vi "FTW-JSON-Variant-Serialize.vi"(0 "Variant":variant, 9 "Pretty Print":bool=TRUE, 11 "error in":errorcluster) -> (4 "JSON String":string, 15 "error out":errorcluster)   [LabVIEW 2015]
uses:
  <vilib>/Utility/Data Type/NI_Data Type.lvlib
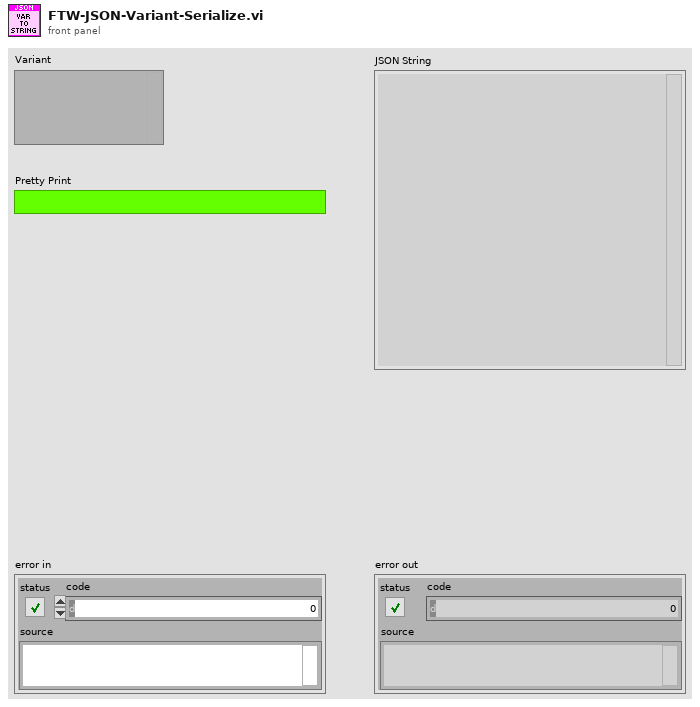
[diagram p1: front panel]
types:
  T1 = cluster{"Include Name":bool, "Indent":i32, "Spaces":i32, "Pretty Print":bool}
  T2 = typedef "NI_Data Type.lvlib/Data Type.ctl" = enum8{"Invalid Type", "Void", "I8", "I16", "I32", "I64", "U8", "U16", "U32", "U64", "Single Float", "Double Float", "Extended Float", "Single Complex", "Double Complex", "Extended Complex", "Enum U8", "Enum U16", "Enum U32", "Enum U64", "Single Float With Unit", "Double Float With Unit", "Extended Float With Unit", "Single Complex with Unit", "Double Complex with Unit", "Extended Complex with Unit", "Boolean", "String", "Path", "Picture", "Tag", "Array", "Cluster", "Variant", "LV Variant", "Waveform", "Timestamp", "Digital Waveform", "Digital Data", "ExpressData", "Refnum", "External Data", "VI", "Poly VI", "LabVIEW Class Instance", "Fixed Point"}
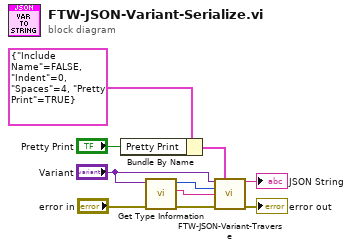
[diagram p0: block diagram]
diagram:
  n1 = Bundle By Name(cluster=T1 {"Include Name"=FALSE, "Indent"=0, "Spaces"=4, "Pretty Print"=TRUE} ("Options"), "Pretty Print"="Pretty Print") -> (w6:T1)
  n2 = call <vilib>:"Get Type Information.vi"("error in (no error)"="error in", "Variant"="Variant") -> ("error out"=w4:errorcluster, "Name"=w2:string, "Type"=w3:T2)  [unwired: 5 in, 2 out]
  n3 = call "FTW-JSON-Variant-Traverse.vi"("Variant"="Variant", "Options"=w6, "Type"=w3, "Name"=w2, "error in"=w4) -> ("JSON String"=→"JSON String":string, "error out"=→"error out":errorcluster)  [unwired: 9 in]
